vi "UDP_send_003.vi"() -> ()   [LabVIEW 2019]
panel:
  in  "Data":dbl(slide) scale=0.0..10.0
  in  "stop":bool
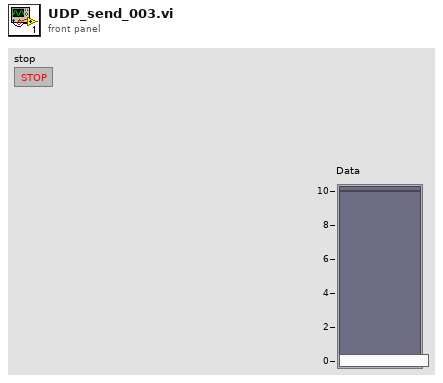
[diagram p1: front panel]
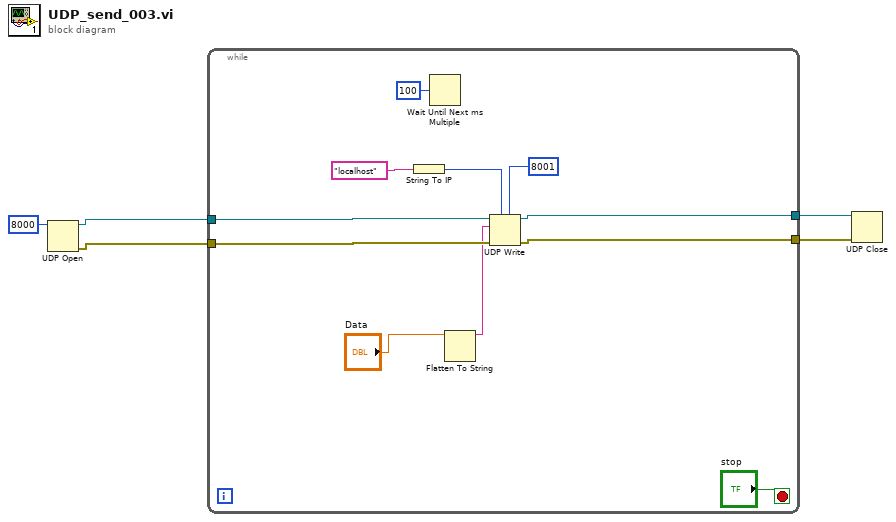
[diagram p0: block diagram]
diagram:
  n1 = UDP Open(11:u16 8000 ("port")) -> (port=w3:refnum<k16>, 0:w5:errorcluster)  [unwired: 4 in, 1 out]
  n2 = while {
    tunnel: w5 -> [w15]
    tunnel: [w14] -> w4
    tunnel: w3 -> [w13]
    tunnel: [w12] -> w2
    stop <- "stop" stop-if-true
    n3 = String To IP(1:"localhost") -> (0:w8:u32)
    n4 = Wait Until Next ms Multiple(millisecond multiple=u32 100) -> ()  [unwired: 1 out]
    n5 = Flatten To String(anything="Data") -> (data string=w6:string)  [unwired: 3 in, 2 out]
    n6 = UDP Write(address=w8, port or service name=u16 8001, connection ID=w13, data in=w6, 8:w15) -> (error out=w14:errorcluster, 3:w12:refnum<k16>)  [unwired: 1 in]
  }
  n7 = UDP Close(connection ID=w2, 8:w4) -> ()  [unwired: 2 out]
